vi "RVC Skew Matrix.vi"() -> ()   [LabVIEW 2013]
uses:
  <vilib>/Analysis/baseanly.llb/Real A x B.vi
  <vilib>/Analysis/7linalg.llb/Create Special Real Matrix.vi
  <vilib>/Analysis/Matrix/Numeric/Subtract/Subtract - RM,RM.vi
  <vilib>/robotics/Kinematics/NI_Kinematics.lvlib
  <vilib>/Analysis/NI_AALBase.lvlib
  <vilib>/Analysis/NI_AALPro.lvlib
  <vilib>/Analysis/Matrix/NI_Matrix.lvlib
panel:
  out "final pose":picture
  out "T1 2":picture
  out "difference":dbl[](array[numeric])
  out "T1":picture
  out "Commutative Rdelta":picture
  out "Rdelta":picture
  out "skew vector out":dbl[](array[numeric]) format="%.4g"
  out "matrix difference":picture
  out "Commutative Rdelta":picture
  out "Rdelta":picture
  out "vector out":dbl[](array[numeric])=[1.0, 2.0, 3.0]
  out "matrix":picture
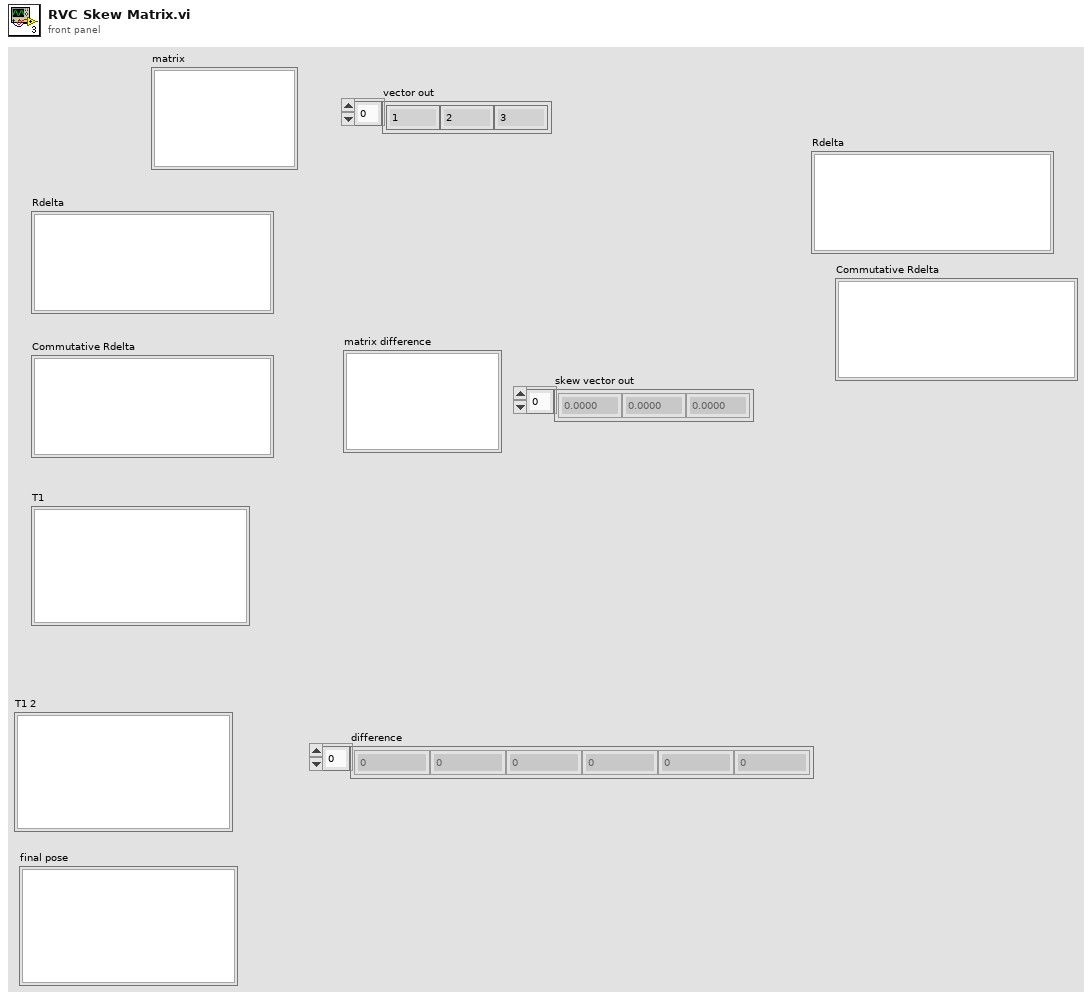
[diagram p1: front panel]
types:
  T1 = typedef "NI_Matrix.lvlib/RealMatrix.ctl" = dbl[][]
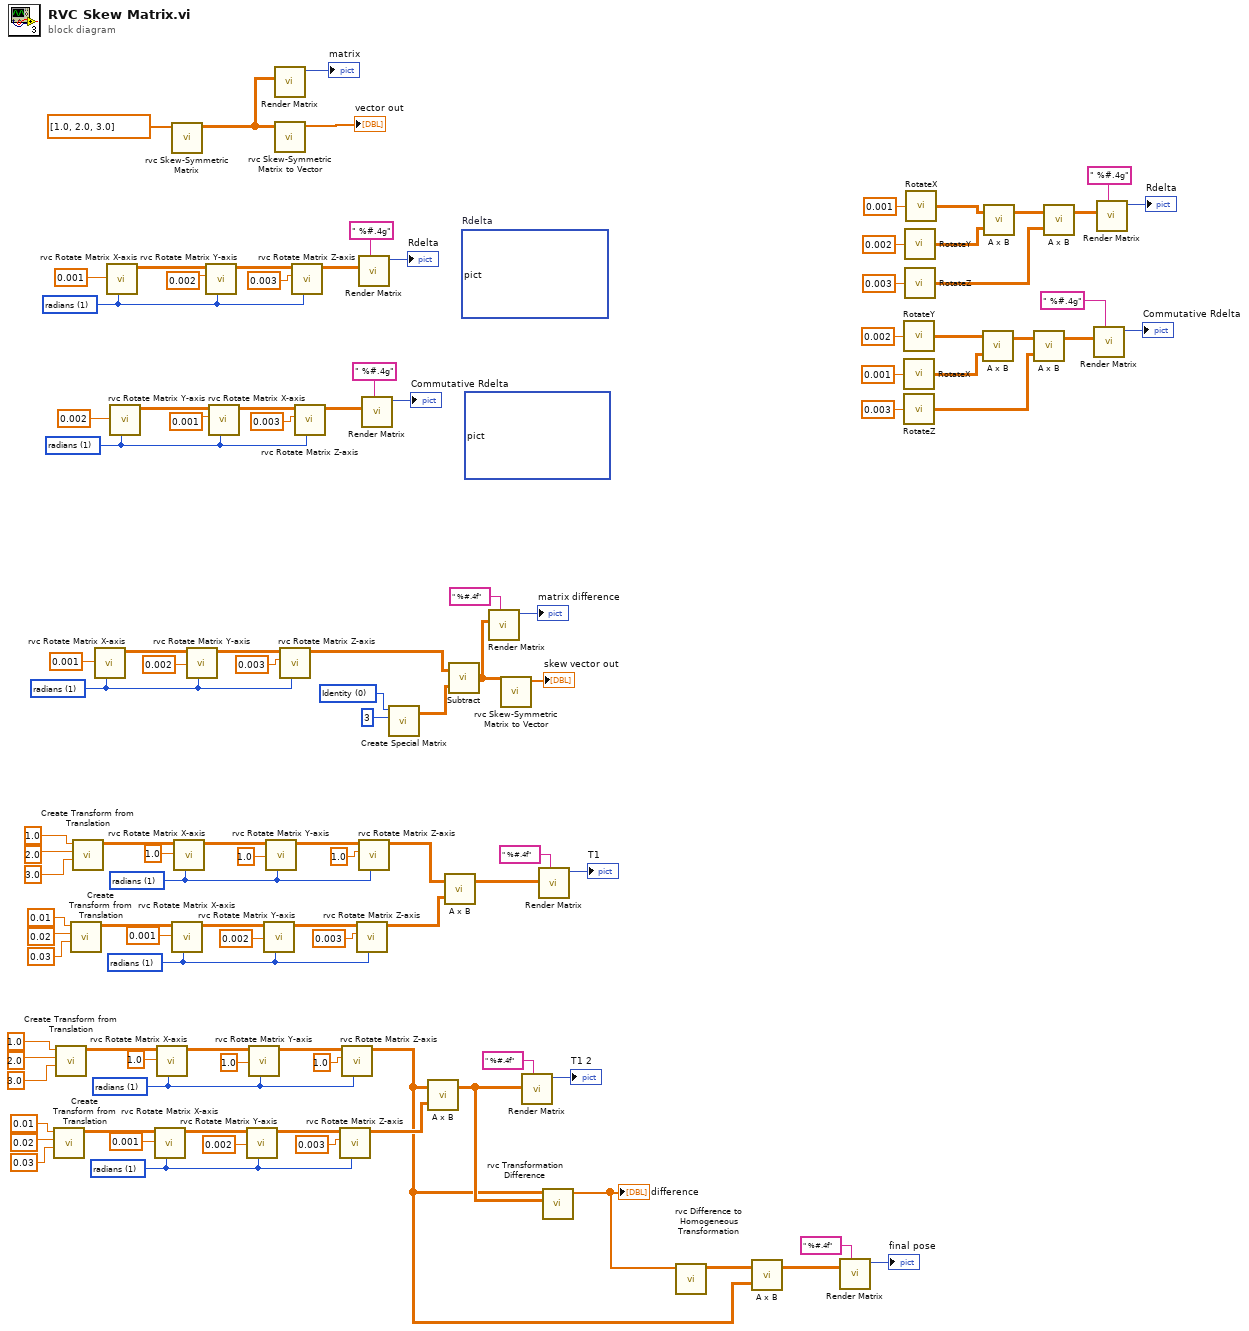
[diagram p0: block diagram]
diagram:
  w19 = u16 1 items=["degree", "radians"] ("angle unit")
  w16 = u16 1 items=["degree", "radians"] ("angle unit")
  w45 = u16 1 items=["degree", "radians"] ("angle unit")
  w48 = u16 1 items=["degree", "radians"] ("angle unit")
  (unwired) picture bytes[526] ("Commutative Rdelta")
  (unwired) picture bytes[526]  # Rdelta
  w64 = u16 1 items=["degree", "radians"] ("angle unit")
  w73 = u16 1 items=["degree", "radians"] ("angle unit")
  w74 = u16 1 items=["degree", "radians"] ("angle unit")
  w88 = 0 items=["Identity", "Diagonal", "Toeplitz", "Vandermonde", "Companion", "Hankel", "Hadamard", "Wilkinson", "Hilbert", "Inverse Hilbert", "Rosser", "Pascal"] ("matrix type")
  n1 = call <vilib>:"Create Transform from Translation.vi"("z"=0.03 ("Numeric"), "y"=0.02 ("Numeric"), "x"=0.01 ("Numeric")) -> ("transform"=w18:T1)  [unwired: 8 in]
  n2 = call <vilib>:"Create Transform from Translation.vi"("z"=3.0 ("Numeric"), "y"=2.0 ("Numeric"), "x"=1.0 ("Numeric")) -> ("transform"=w17:T1)  [unwired: 8 in]
  n3 = call <vilib>:"Create Transform from Translation.vi"("z"=0.03 ("Numeric"), "y"=0.02 ("Numeric"), "x"=0.01 ("Numeric")) -> ("transform"=w46:T1)  [unwired: 8 in]
  n4 = call <vilib>:"Create Transform from Translation.vi"("z"=3.0 ("Numeric"), "y"=2.0 ("Numeric"), "x"=1.0 ("Numeric")) -> ("transform"=w47:T1)  [unwired: 8 in]
  n5 = call "rvc Rotate Matrix X-axis.vi"("angle unit"=w64, "angle"=0.001 ("theta")) -> ("rotation matrix"=w60:T1)  [unwired: 9 in]
  n6 = call "rvc Rotate Matrix X-axis.vi"("angle unit"=w74, "angle"=0.001 ("theta")) -> ("rotation matrix"=w81:T1)  [unwired: 9 in]
  n7 = call "rvc Rotate Matrix Y-axis.vi"("angle unit"=w73, "angle"=0.002 ("theta")) -> ("rotation matrix"=w67:T1)  [unwired: 9 in]
  n8 = call "rvc Rotate Matrix X-axis.vi"("angle unit"=w19, "angle"=0.001 ("theta"), "rotation matrix in"=w18) -> ("rotation matrix"=w23:T1)  [unwired: 8 in]
  n9 = call "rvc Rotate Matrix X-axis.vi"("angle unit"=w16, "angle"=1.0 ("theta"), "rotation matrix in"=w17) -> ("rotation matrix"=w12:T1)  [unwired: 8 in]
  n10 = call "rvc Skew-Symmetric Matrix.vi"("vector"=dbl[] [1.0, 2.0, 3.0]) -> ("output variable"=w109:dbl[][])  [unwired: 10 in]
  n11 = call "rvc Rotate Matrix X-axis.vi"("angle unit"=w45, "angle"=0.001 ("theta"), "rotation matrix in"=w46) -> ("rotation matrix"=w41:T1)  [unwired: 8 in]
  n12 = call "rvc Rotate Matrix X-axis.vi"("angle unit"=w48, "angle"=1.0 ("theta"), "rotation matrix in"=w47) -> ("rotation matrix"=w52:T1)  [unwired: 8 in]
  n13 = call "rvc Rotate Matrix Y-axis.vi"("angle unit"=w64, "angle"=0.002 ("theta"), "rotation matrix in"=w60) -> ("rotation matrix"=w62:T1)  [unwired: 8 in]
  n14 = call "rvc Rotate Matrix Y-axis.vi"("angle unit"=w74, "angle"=0.002 ("theta"), "rotation matrix in"=w81) -> ("rotation matrix"=w79:T1)  [unwired: 8 in]
  n15 = call "rvc Rotate Matrix X-axis.vi"("angle unit"=w73, "angle"=0.001 ("theta"), "rotation matrix in"=w67) -> ("rotation matrix"=w69:T1)  [unwired: 8 in]
  n16 = call "rvc Rotate Matrix Y-axis.vi"("angle unit"=w19, "angle"=0.002 ("theta"), "rotation matrix in"=w23) -> ("rotation matrix"=w21:T1)  [unwired: 8 in]
  n17 = call "rvc Rotate Matrix Y-axis.vi"("angle unit"=w16, "angle"=1.0 ("theta"), "rotation matrix in"=w12) -> ("rotation matrix"=w14:T1)  [unwired: 8 in]
  n18 = call "rvc Rotate Matrix Y-axis.vi"("angle unit"=w45, "angle"=0.002 ("theta"), "rotation matrix in"=w41) -> ("rotation matrix"=w43:T1)  [unwired: 8 in]
  n19 = call "rvc Rotate Matrix Y-axis.vi"("angle unit"=w48, "angle"=1.0 ("theta"), "rotation matrix in"=w52) -> ("rotation matrix"=w50:T1)  [unwired: 8 in]
  n20 = call "Render Matrix.vi"("A"=w109) -> ("picture out"=→"matrix":picture)  [unwired: 10 in]
  n21 = call "rvc Skew-Symmetric Matrix to Vector.vi"("output variable in"=w109) -> ("output variable out"=→"vector out":dbl[])  [unwired: 10 in]
  n22 = call "rvc Rotate Matrix Z-axis.vi"("angle unit"=w64, "angle"=0.003 ("theta"), "rotation matrix in"=w62) -> ("rotation matrix"=w58:T1)  [unwired: 8 in]
  n23 = call "rvc Rotate Matrix Z-axis.vi"("angle unit"=w74, "angle"=0.003 ("theta"), "rotation matrix in"=w79) -> ("rotation matrix"=w75:T1)  [unwired: 8 in]
  n24 = call "rvc Rotate Matrix Z-axis.vi"("angle unit"=w73, "angle"=0.003 ("theta"), "rotation matrix in"=w69) -> ("rotation matrix"=w72:T1)  [unwired: 8 in]
  n25 = call "rvc Rotate Matrix Z-axis.vi"("angle unit"=w19, "angle"=0.003 ("theta"), "rotation matrix in"=w21) -> ("rotation matrix"=w30:T1)  [unwired: 8 in]
  n26 = call "rvc Rotate Matrix Z-axis.vi"("angle unit"=w16, "angle"=1.0 ("theta"), "rotation matrix in"=w14) -> ("rotation matrix"=w2:T1)  [unwired: 8 in]
  n27 = call "rvc Rotate Matrix Z-axis.vi"("angle unit"=w45, "angle"=0.003 ("theta"), "rotation matrix in"=w43) -> ("rotation matrix"=w34:T1)  [unwired: 8 in]
  n28 = call "Render Matrix.vi"("format string"=" %#.4g", "A"=w75) -> ("picture out"=→"Rdelta":picture)  [unwired: 9 in]
  n29 = call "rvc Rotate Matrix Z-axis.vi"("angle unit"=w48, "angle"=1.0 ("theta"), "rotation matrix in"=w50) -> ("rotation matrix"=w33:T1)  [unwired: 8 in]
  n30 = call "Render Matrix.vi"("format string"=" %#.4g", "A"=w72) -> ("picture out"=→"Commutative Rdelta":picture)  [unwired: 9 in]
  n31 = call-poly <vilib>:"Create Special Matrix.vi"("matrix type"=w88, "matrix size"=3) -> ("Special Matrix"=w87:T1)  [unwired: 3 in, 1 out]
  n32 = call-poly <vilib>:"A x B.vi"("B"=w30, "A"=w2) -> ("A x B"=w31:T1)  [unwired: 1 out]
  n33 = call-poly <vilib>:"A x B.vi"("B"=w34, "A"=w33) -> ("A x B"=w32:T1)  [unwired: 1 out]
  n34 = call-poly <vilib>:"Subtract.vi"("Real Matrix B"=w87, "Real Matrix A"=w58) -> ("A - B"=w84:T1)
  n35 = call "Render Matrix.vi"("format string"=" %#.4f", "A"=w84) -> ("picture out"=→"matrix difference":picture)  [unwired: 9 in]
  n36 = call "rvc Skew-Symmetric Matrix to Vector.vi"("output variable in"=w84) -> ("output variable out"=→"skew vector out":dbl[])  [unwired: 10 in]
  n37 = call "Render Matrix.vi"("format string"=" %#.4f", "A"=w31) -> ("picture out"=→"T1 2":picture)  [unwired: 9 in]
  n38 = call "Render Matrix.vi"("format string"=" %#.4f", "A"=w32) -> ("picture out"=→"T1":picture)  [unwired: 9 in]
  n39 = call "rvc Transformation Difference.vi"("Final transformation"=w31, "Initial transformation"=w2) -> ("Difference"=w6:dbl[])  [unwired: 9 in]
  "difference" <- w6
  n40 = call "rvc Difference to Homogeneous Transformation.vi"("Difference"=w6) -> ("Matrix Transformation"=w1:T1)  [unwired: 10 in]
  n41 = call-poly <vilib>:"A x B.vi"("B"=w2, "A"=w1) -> ("A x B"=w3:T1)  [unwired: 1 out]
  n42 = call "Render Matrix.vi"("format string"=" %#.4f", "A"=w3) -> ("picture out"=→"final pose":picture)  [unwired: 9 in]
  n43 = call <vilib>:"RotateY.vi"("theta"=0.002) -> ("rotation matrix"=w93:T1)
  n44 = call <vilib>:"RotateX.vi"("theta"=0.001) -> ("rotation matrix"=w92:T1)
  n45 = call <vilib>:"RotateZ.vi"("theta"=0.003) -> ("rotation matrix"=w94:T1)
  n46 = call <vilib>:"RotateY.vi"("theta"=0.002) -> ("rotation matrix"=w106:T1)
  n47 = call <vilib>:"RotateZ.vi"("theta"=0.003) -> ("rotation matrix"=w105:T1)
  n48 = call <vilib>:"RotateX.vi"("theta"=0.001) -> ("rotation matrix"=w107:T1)
  n49 = call-poly <vilib>:"A x B.vi"("B"=w92, "A"=w93) -> ("A x B"=w95:T1)  [unwired: 1 out]
  n50 = call-poly <vilib>:"A x B.vi"("B"=w106, "A"=w107) -> ("A x B"=w104:T1)  [unwired: 1 out]
  n51 = call-poly <vilib>:"A x B.vi"("B"=w94, "A"=w95) -> ("A x B"=w86:T1)  [unwired: 1 out]
  n52 = call-poly <vilib>:"A x B.vi"("B"=w105, "A"=w104) -> ("A x B"=w100:T1)  [unwired: 1 out]
  n53 = call "Render Matrix.vi"("format string"=" %#.4g", "A"=w86) -> ("picture out"=→"Commutative Rdelta":picture)  [unwired: 9 in]
  n54 = call "Render Matrix.vi"("format string"=" %#.4g", "A"=w100) -> ("picture out"=→"Rdelta":picture)  [unwired: 9 in]
